vi "Slow to Item.vi"(8 "error in (no error)":errorcluster, 10 "Position Change":i32, 11 "ScrollingList in":refnum<class "ScrollingList.lvclass">) -> (0 "error out":errorcluster, 3 "ScrollingList out":refnum<class "ScrollingList.lvclass">)   [LabVIEW 2020, in "ScrollingList.lvclass"]
uses:
  ScrollingList.lvclass
  ScrollingList.lvclass/ScrollingList.ctl
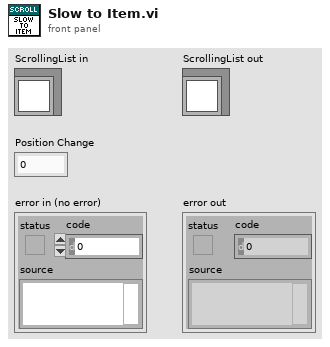
[diagram p1: front panel]
types:
  T1 = typedef "ScrollingList.lvclass/State Data.ctl" = cluster{"Timeout":i32, "Time":timestamp, "Y":i32, "Origin:Top":i16, "Rate":dbl, "ListItems":string[], "Item Height":i32, "Max Height":i32}
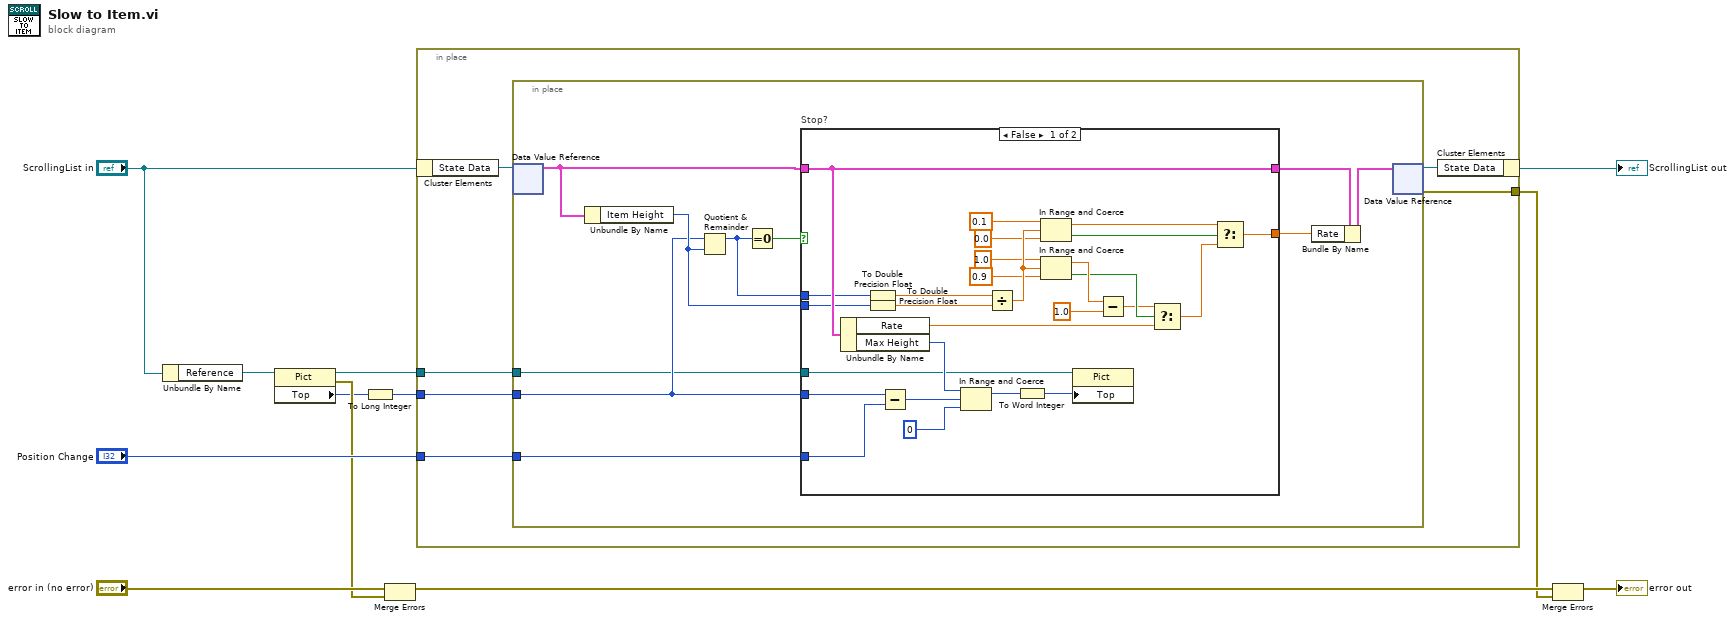
[diagram p0: block diagram]
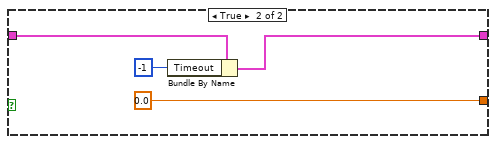
[diagram p2: hidden frame]
diagram:
  n1 = Unbundle By Name("ScrollingList in") -> ("Reference"=w7:refnum<vi>)
  n2 = property class="Pict"(reference=w7) -> (reference out=w4:refnum<vi>, error out=w3:errorcluster, "Top"=w2:i16)  [unwired: 1 in]
  n3 = To Long Integer(number=w2) -> (32bit integer=w10:i32)
  n4 = Merge Errors("error in (no error)", w3) -> (w9:errorcluster)
  n5 = in-place {
    in-place-border: w10 -> [w16]
    in-place-border: "Position Change" -> [w15]
    in-place-border: w4 -> [w14]
    in-place-border: [w13] -> w5
    n6 = in-place-cluster #1("ScrollingList in") -> ("State Data"=w18:refnum<data-value>)
    n7 = in-place {
      in-place-border: w16 -> [w20]
      in-place-border: w15 -> [w21]
      in-place-border: w14 -> [w19]
      n8 = in-place-dvr #2(w18) -> (w28:T1)  [unwired: 1 out]
      n9 = Unbundle By Name(w28) -> ("Item Height"=w22:i32)
      n10 = Quotient & Remainder(x=w20, y=w22) -> (x-y*floor(x/y)=w23:i32)  [unwired: 1 out]
      n11 = Equal To 0?(x=w23) -> (x = 0?=w24:bool)
      n12 = case "Stop?" shown="False" w24 {
        tunnel: w28 -> [w50 w58]
        tunnel: [w50 w57] -> w26
        tunnel: w19 -> [w52 _]
        tunnel: w20 -> [w51 _]
        tunnel: w21 -> [w49 _]
        tunnel: [w31 0.0 ("x")] -> w27
        tunnel: w22 -> [w37 _]
        tunnel: w23 -> [w36 _]
        frame False {
          n13 = Unbundle By Name(w50) -> ("Rate"=w33:dbl, "Max Height"=w54:i32)
          n14 = To Double Precision Float(number=w36) -> (double precision float=w38:dbl)
          n15 = To Double Precision Float(number=w37) -> (double precision float=w39:dbl)
          n16 = Subtract(x=w51, y=w49) -> (x-y=w30:i32)
          n17 = In Range and Coerce(upper limit=w54, x=w30, lower limit=0) -> (coerced(x)=w29:i32)  [unwired: 1 out]
          n18 = Divide(x=w38, y=w39) -> (x/y=w44:dbl)
          n19 = To Word Integer(number=w29) -> (16bit integer=w55:i16)
          n20 = In Range and Coerce(upper limit=0.1, x=w44, lower limit=0.0) -> (coerced(x)=w45:dbl, In Range?=w46:bool)
          n21 = In Range and Coerce(upper limit=1.0, x=w44, lower limit=0.9) -> (coerced(x)=w47:dbl, In Range?=w35:bool)
          n22 = property on="Property Node" class="Pict"(reference=w52, "Top"=w55) -> ()  [unwired: 1 in, 2 out]
          n23 = Subtract(x=w47, y=1.0 ("x")) -> (x-y=w34:dbl)
          n24 = Select(t=w34, s=w35, f=w33) -> (s? t:f=w32:dbl)
          n25 = Select(t=w45, s=w46, f=w32) -> (s? t:f=w31:dbl)
        }
        frame True {
          n26 = Bundle By Name(cluster=w58, "Timeout"=-1) -> (w57:T1)
        }
      }
      n27 = Bundle By Name(cluster=w26, "Rate"=w27) -> (w25:T1)
      n28 = in-place-dvr #2(w25) -> (w17:refnum<data-value>, w13:errorcluster)
    }
    n29 = in-place-cluster #1("State Data"=w17) -> (→"ScrollingList out":refnum<class "ScrollingList.lvclass">)
  }
  n30 = Merge Errors(w9, w5) -> (→"error out":errorcluster)
